vi "Get UI VI Reference.vi"(8 "error in (no error)":errorcluster, 11 "Game Mode in":refnum<class "Game Mode.lvclass">) -> (0 "error out":errorcluster, 2 "VI Refnum":refnum<vi>, 3 "Game Mode out":refnum<class "Game Mode.lvclass">)   [LabVIEW 2017, in "Game Mode.lvclass"]
uses:
  Game Mode.lvclass
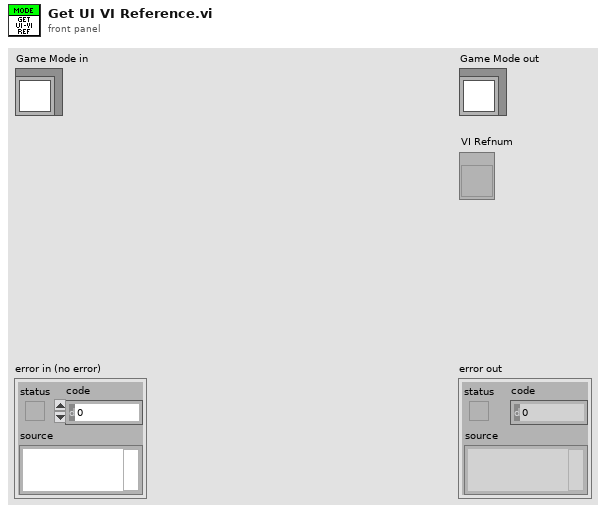
[diagram p1: front panel]
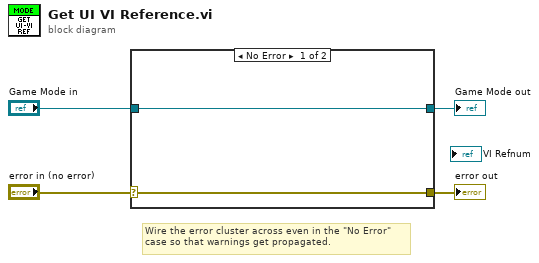
[diagram p0: block diagram]
diagram:
  # "Wire the error cluster across even in the \"No Error\"\ncase so that warnings get propagated."
  n1 = case shown="No Error" "error in (no error)" {
    selector: "error in (no error)" -> [w5 w8]
    tunnel: [w5 w8] -> w3
    tunnel: [w6 w7] -> w1
    tunnel: "Game Mode in" -> [w6 w7]
    frame No Error {
    }
    frame Error {
    }
  }
  "error out" <- w3
  "Game Mode out" <- w1
